vi "uc480_SubVI_Example_GetDefault_Timing.vi"(0 ".NET (Reference)":refnum<k24>, 11 "Error In":errorcluster) -> (6 "Pixelclock":i32, 8 "Exposure time":dbl, 10 "Framerate":dbl, 15 "Error Out":errorcluster)   [LabVIEW 2015]
uses:
  C:/Program Files/Thorlabs/Scientific Imaging/DCx Camera Support/Develop/DotNet/uc480DotNet.dll
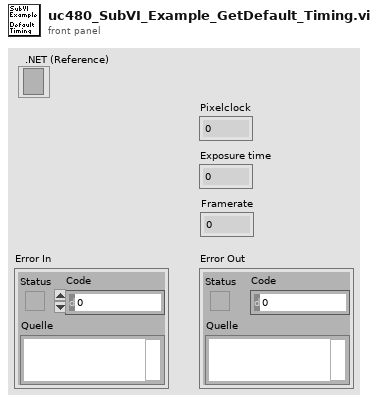
[diagram p1: front panel]
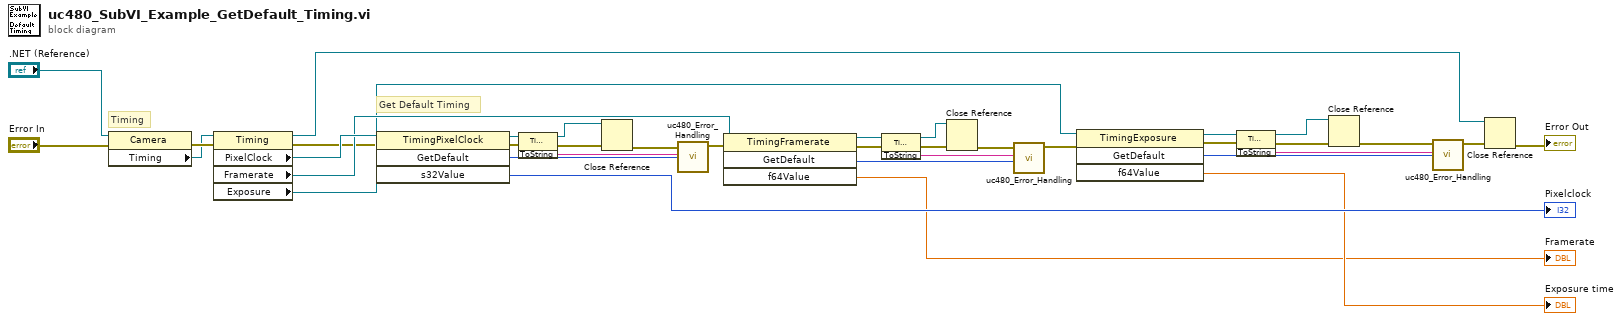
[diagram p0: block diagram]
diagram:
  # "Get Default Timing"
  # "Timing"
  n1 = property class="Camera"(reference=".NET (Reference)", error in="Error In") -> (error out=w35:errorcluster, "Timing"=w34:refnum<k24>)  [unwired: 1 out]
  n2 = property class="Timing"(reference=w34, error in=w35) -> (reference out=w10:refnum<k24>, error out=w13:errorcluster, "PixelClock"=w33:refnum<k24>, "Framerate"=w18:refnum<k24>, "Exposure"=w16:refnum<k24>)
  n3 = invoke class="TimingPixelClock" method="GetDefault"(reference=w33, error in=w13) -> (reference out=w31:refnum<k24>, error out=w30:errorcluster, "GetDefault"=w28:i32, "s32Value"=→"Pixelclock":i32)  [unwired: 2 in]
  n4 = invoke class="TimingPixelClock" method="ToString"(reference=w31, error in=w30) -> (reference out=w2:refnum<k24>, error out=w3:errorcluster, "ToString"=w29:string)  [unwired: 1 in]
  n5 = Close Reference(reference=w2, error in (no error)=w3) -> (error out=w1:errorcluster)
  n6 = call "uc480_Error_Handling.vi"("Error Code"=w28, "Error String"=w29, "Error In"=w1) -> ("Error Out"=w19:errorcluster)  [unwired: 8 in]
  n7 = invoke class="TimingFramerate" method="GetDefault"(reference=w18, error in=w19) -> (reference out=w27:refnum<k24>, error out=w26:errorcluster, "GetDefault"=w24:i32, "f64Value"=→"Framerate":dbl)  [unwired: 2 in]
  n8 = invoke class="TimingFramerate" method="ToString"(reference=w27, error in=w26) -> (reference out=w4:refnum<k24>, error out=w6:errorcluster, "ToString"=w25:string)  [unwired: 1 in]
  n9 = Close Reference(reference=w4, error in (no error)=w6) -> (error out=w5:errorcluster)
  n10 = call "uc480_Error_Handling.vi"("Error Code"=w24, "Error String"=w25, "Error In"=w5) -> ("Error Out"=w17:errorcluster)  [unwired: 8 in]
  n11 = invoke class="TimingExposure" method="GetDefault"(reference=w16, error in=w17) -> (reference out=w23:refnum<k24>, error out=w22:errorcluster, "GetDefault"=w20:i32, "f64Value"=→"Exposure time":dbl)  [unwired: 2 in]
  n12 = invoke class="TimingExposure" method="ToString"(reference=w23, error in=w22) -> (reference out=w7:refnum<k24>, error out=w9:errorcluster, "ToString"=w21:string)  [unwired: 1 in]
  n13 = Close Reference(reference=w7, error in (no error)=w9) -> (error out=w8:errorcluster)
  n14 = call "uc480_Error_Handling.vi"("Error Code"=w20, "Error String"=w21, "Error In"=w8) -> ("Error Out"=w12:errorcluster)  [unwired: 8 in]
  n15 = Close Reference(reference=w10, error in (no error)=w12) -> (error out=→"Error Out":errorcluster)
